vi "LDO Array Data.vi"(0 "PLC Data In":T1, 1 "Burner ON Ref":refnum<vi>, 2 "0.8 ML Ref":refnum<vi>, 3 "1.1 ML Ref":refnum<vi>, 5 "Gas Data":T7, 7 "Inficon Data Input":T6, 8 "1.33 ML Ref":refnum<vi>, 9 "Ultramat 23":string[][](array[string]), 10 "Start recording data":refnum<vi>, 11 "error in (no error)":errorcluster, 12 "Event Booleans in":T5, 13 "Pilot Rate (BTU/hr)":dbl=600.0) -> (4 "PLC Data Out":T1, 6 "LDO Array":string[][](array[string]), 14 "Event Booleans out":T5, 15 "error out":errorcluster)   [LabVIEW 2020]
uses:
  Modbus/Modbus PLC Data All.ctl
  Modbus/Modbus FVIR Control.ctl
  Modbus/Modbus LDO Control.ctl
  WritingDataFile/Data to Save.ctl
  Modbus/Modbus Gas Meter Data.ctl
  Drivers/Alicat LabVIEW Drivers 2v1/Sub-VIs/Data Cluster.ctl
  Drivers/Alicat LabVIEW Drivers 2v1/Sub-VIs/Units of Measure.ctl
  Drivers/Inficon Transmitter/Type Definitions/Inficon Data.ctl
  Event Booleans.ctl
panel:
  out "Burner ON":bool
  # "Natural Gas"
  # "Propane"
  # "Totalizer Timer"
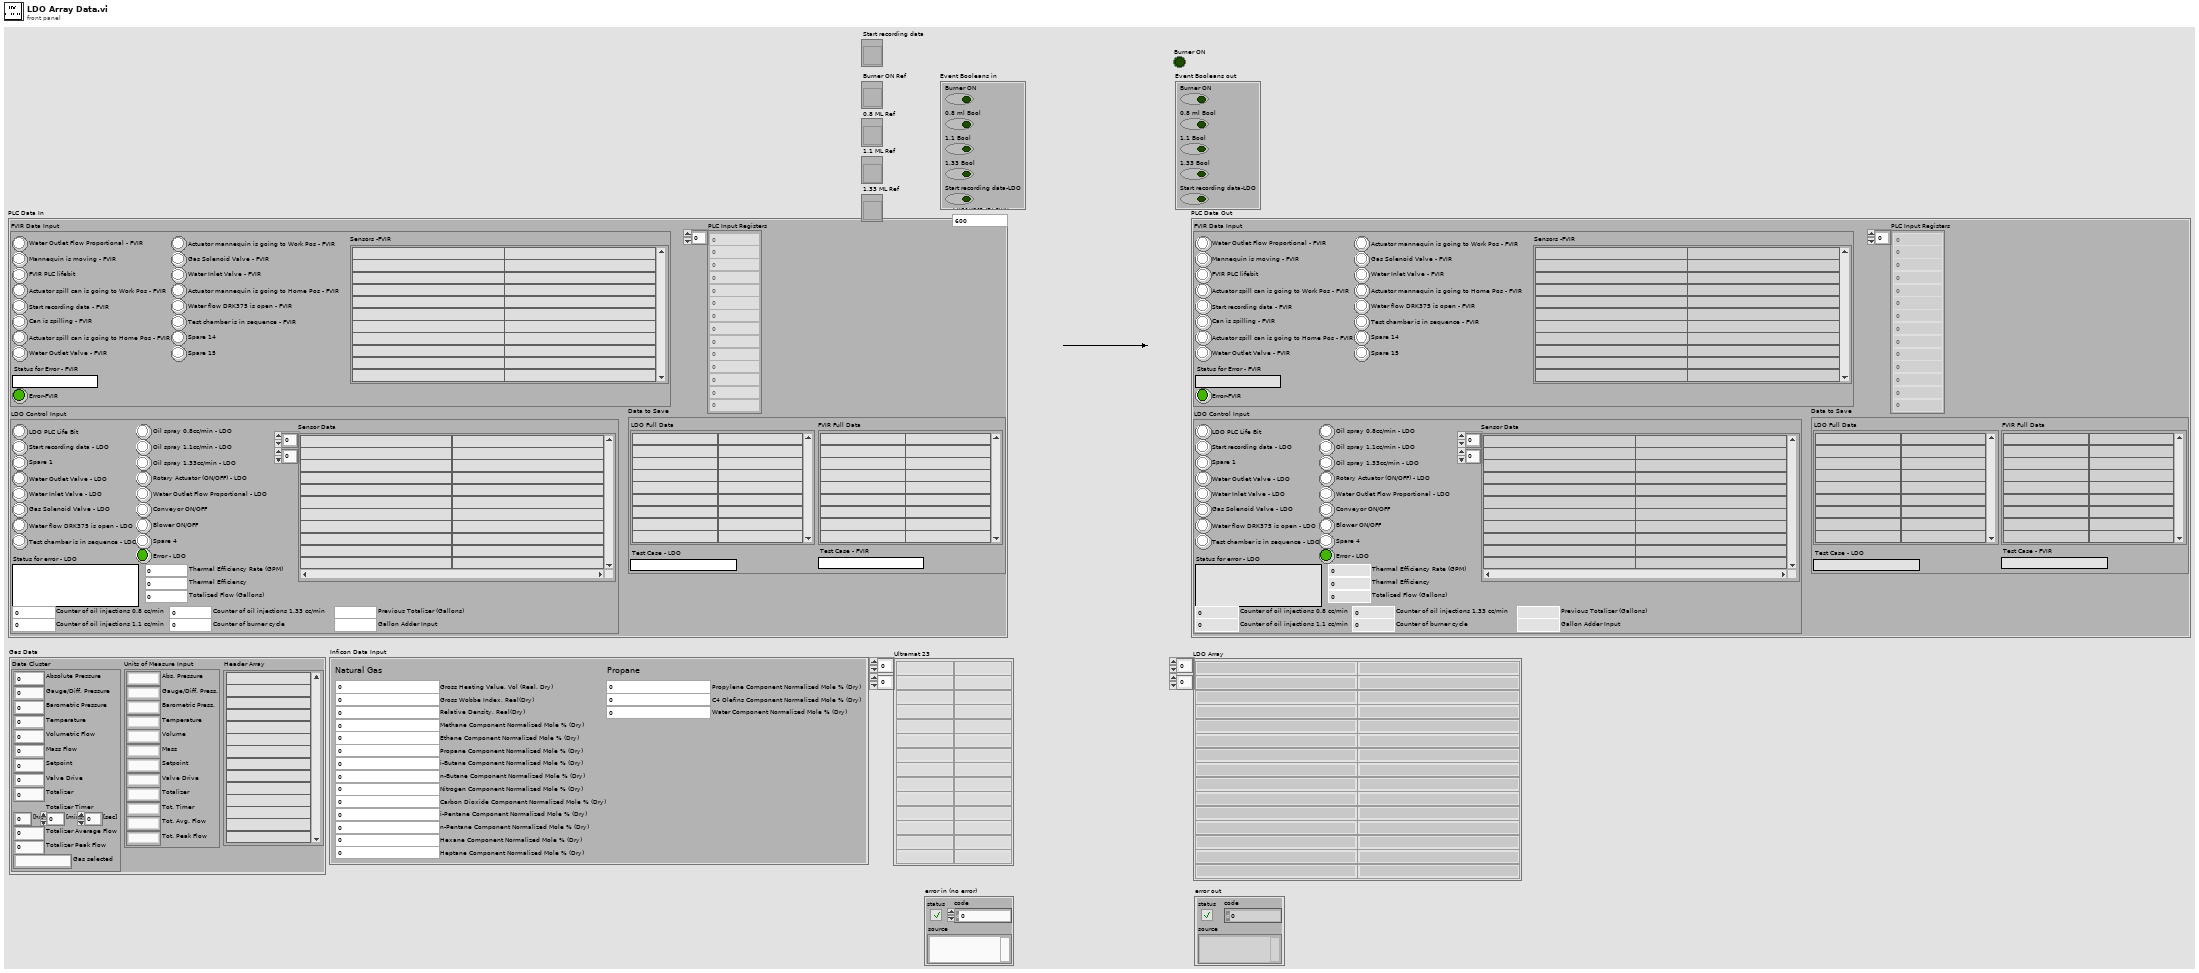
[diagram p1: front panel]
types:
  T1 = typedef "Modbus PLC Data All.ctl" = cluster{"FVIR Data Input":T2, "LDO Control Input":T3, "PLC Input Registers":i16[], "Data to Save":T4}
  T2 = typedef "Modbus FVIR Control.ctl" = cluster{"Spare 15":bool, "Spare 14":bool, "Actuator mannequin is going to Work Pos - FVIR":bool, "Actuator mannequin is going to Home Pos - FVIR":bool, "Test chamber is in sequence - FVIR ":bool, "Water flow DRK375 is open - FVIR":bool, "Gas Solenoid Valve - FVIR":bool, "Water Inlet Valve - FVIR":bool, "Water Outlet Flow Proportional - FVIR":bool, "Start recording data - FVIR":bool, "Actuator spill can is going to Work Pos - FVIR":bool, "Actuator spill can is going to Home Pos - FVIR":bool, "Water Outlet Valve - FVIR":bool, "Can is spilling - FVIR":bool, "Mannequin is moving - FVIR":bool, "FVIR PLC lifebit":bool, "Status for Error - FVIR":string, "Error-FVIR":bool, "Sensors -FVIR":string[][]}
  T3 = typedef "Modbus LDO Control.ctl" = cluster{"LDO PLC Life Bit":bool, "Start recording data - LDO":bool, "Spare 1":bool, "Water Outlet Valve - LDO":bool, "Water Inlet Valve - LDO":bool, "Gas Solenoid Valve - LDO":bool, "Water flow DRK375 is open - LDO":bool, "Test chamber is in sequence - LDO":bool, "Oil spray 0.8cc/min - LDO":bool, "Oil spray 1.1cc/min - LDO":bool, "Oil spray 1.33cc/min - LDO":bool, "Rotary Actuator (ON/OFF) - LDO":bool, "Water Outlet Flow Proportional - LDO":bool, "Conveyor ON/OFF":bool, "Blower ON/OFF":bool, "Spare 4":bool, "Status for error - LDO":string, "Error - LDO":bool, "Sensor Data":string[][], "Thermal Efficiency Rate (GPM)":dbl, "Thermal Efficiency":dbl, "Totalized Flow (Gallons)":dbl, "Counter of oil injections 1.33 cc/min":u16, "Counter of burner cycle":u16, "Counter of oil injections 1.1 cc/min":u16, "Counter of oil injections 0.8 cc/min":u16, "Previous Totalizer (Gallons)":dbl, "Gallon Adder Input":dbl}
  T4 = typedef "Data to Save.ctl" = cluster{"LDO Full Data":string[][], "FVIR Full Data":string[][], "Test Case - FVIR":string, "Test Case - LDO":string}
  T5 = typedef "Event Booleans.ctl" = cluster{"Burner ON":bool, "0.8 ml Bool":bool, "1.1 Bool":bool, "1.33 Bool":bool, "Start recording data-LDO":bool}
  T6 = typedef "Inficon Data.ctl" = cluster{"Gross Heating Value, Vol (Real, Dry)":dbl, "Nitrogen Component Normalized Mole % (Dry)":dbl, "Methane Component Normalized Mole % (Dry)":dbl, "Carbon Dioxide Component Normalized Mole % (Dry)":dbl, "Ethane Component Normalized Mole % (Dry)":dbl, "Propane Component Normalized Mole % (Dry)":dbl, "i-Pentane Component Normalized Mole % (Dry)":dbl, "i-Butane Component Normalized Mole % (Dry)":dbl, "n-Butane Component Normalized Mole % (Dry)":dbl, "n-Pentane Component Normalized Mole % (Dry)":dbl, "Hexane Component Normalized Mole % (Dry)":dbl, "Heptane Component Normalized Mole % (Dry)":dbl, "Gross Wobbe Index, Real(Dry)":dbl, "Relative Density, Real(Dry)":dbl, "Propylene Component Normalized Mole % (Dry)":dbl, "C4 Olefins Component Normalized Mole % (Dry)":dbl, "Water Component Normalized Mole % (Dry)":dbl}
  T7 = typedef "Modbus Gas Meter Data.ctl" = cluster{"Data Cluster":T8, "Units of Measure Input":T9, "Header Array":string[]}
  T8 = typedef "Data Cluster.ctl" = cluster{"Absolute Pressure":dbl, "Gauge/Diff. Pressure":dbl, "Barometric Pressure":dbl, "Temperature":dbl, "Volumetric Flow":dbl, "Mass Flow":dbl, "Setpoint":dbl, "Valve Drive":dbl, "Totalizer":dbl, "[hr]":dbl, "[min]":dbl, "[sec]":dbl, "Totalizer Average Flow":dbl, "Totalizer Peak Flow":dbl, "Gas selected":string}
  T9 = typedef "Units of Measure.ctl" = cluster{"Abs. Pressure":string, "Gauge/Diff. Press.":string, "Barometric Press.":string, "Temperature":string, "Volume":string, "Mass":string, "Setpoint":string, "Valve Drive":string, "Totalizer":string, "Tot. Timer":string, "Tot. Avg. Flow":string, "Tot. Peak Flow":string}
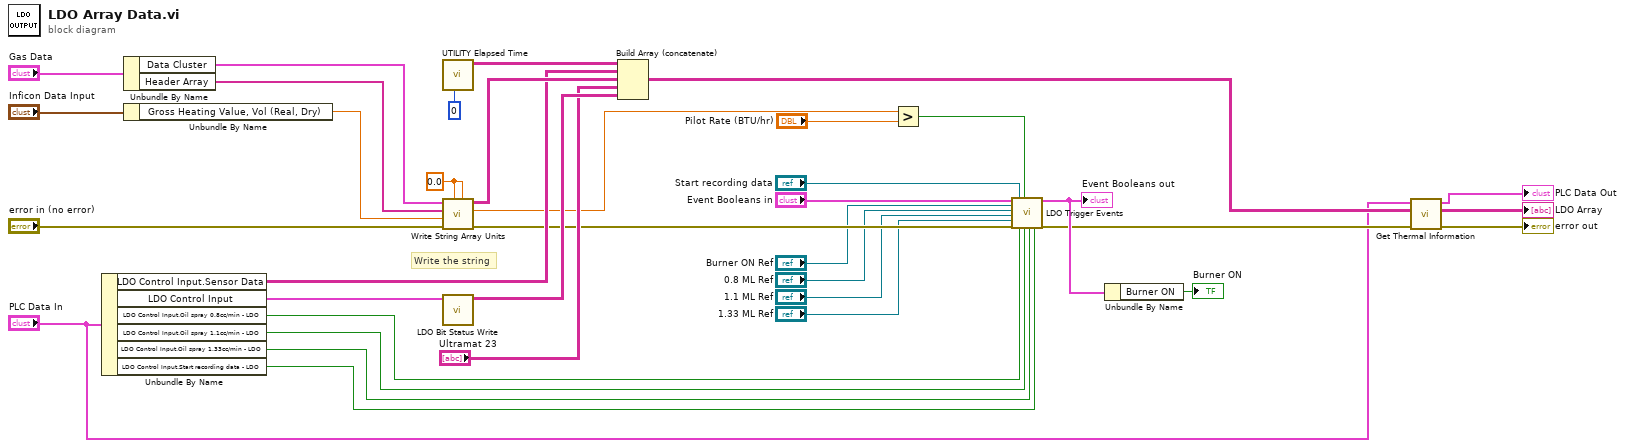
[diagram p0: block diagram]
diagram:
  w30 = 0.0 ("HHV_1")
  # "Write the string"
  n1 = Unbundle By Name("PLC Data In") -> ("LDO Control Input.Sensor Data"=w29:string[][], "LDO Control Input"=w28:T3, "LDO Control Input.Oil spray 0.8cc/min - LDO"=w18:bool, "LDO Control Input.Oil spray 1.1cc/min - LDO"=w17:bool, "LDO Control Input.Oil spray 1.33cc/min - LDO"=w16:bool, "LDO Control Input.Start recording data - LDO"=w1:bool)
  n2 = Unbundle By Name("Gas Data") -> ("Data Cluster"=w26:T8, "Header Array"=w25:string[])
  n3 = Unbundle By Name("Inficon Data Input") -> ("Gross Heating Value, Vol (Real, Dry)"=w23:dbl)
  n4 = call "UTILITY Elapsed Time.vi"("precision (6)"=i16 0) -> ("Total Array"=w35:string[][])  [unwired: 6 in, 4 out]
  n5 = call "Write String Array Units.vi"("Total_1"=w30, "HHV_1"=w30, "Error In"="error in (no error)", "Gross Heating Value, Vol (Real, Dry)"=w23, "Header Array"=w25, "Data Cluster"=w26) -> ("Error Out"=w19:errorcluster, "Gas Rate (BTU/hr)"=w20:dbl, "String Data"=w31:string[][])  [unwired: 3 in]
  n6 = call "LDO Bit Status Write.vi"("LDO Control Input"=w28) -> ("Bit Status"=w34:string[][])  [unwired: 9 in, 1 out]
  n7 = Build Array (concatenate)(w35, w29, w31, "Ultramat 23", w34) -> (w7:string[][])
  n8 = Greater?(x=w20, y="Pilot Rate (BTU/hr)") -> (0:w22:bool)
  n9 = call "LDO Trigger Events.vi"("Event Booleans in"="Event Booleans in", "Burner ON Ref"="Burner ON Ref", "0.8 ML Ref"="0.8 ML Ref", "1.1 ML Ref"="1.1 ML Ref", "1.33 ML Ref"="1.33 ML Ref", "error in"=w19, "Start recording data"="Start recording data", "Oil spray 0.8cc/min - LDO"=w18, "Burner ON"=w22, "Oil spray 1.1cc/min - LDO"=w17, "Oil spray 1.33cc/min - LDO"=w16, "Start recording data-LDO"=w1) -> ("Event Booleans out"=w10:T5, "error out"=w8:errorcluster)  [unwired: 6 in]
  "Event Booleans out" <- w10
  n10 = Unbundle By Name(w10) -> ("Burner ON"=→"Burner ON":bool)
  n11 = call "Get Thermal Information.vi"("error in"=w8, "LDO Input"=w7, "PLC Data In"="PLC Data In") -> ("error out"=→"error out":errorcluster, "LDO Output"=→"LDO Array":string[][], "PLC Data Out"=→"PLC Data Out":T1)  [unwired: 6 in]
